vi "SSH_TUNNEL_Close.vi"(8 "error in (no error)":errorcluster, 11 "SSH_TUNNEL in":refnum<class "SSH_TUNNEL.lvclass">) -> (0 "error out":errorcluster, 3 "SSH_TUNNEL out":refnum<class "SSH_TUNNEL.lvclass">)   [LabVIEW 2018, in "SSH_TUNNEL.lvclass"]
uses:
  SSH_TUNNEL.lvclass
  SSH_TUNNEL.lvclass/SSH_TUNNEL.ctl
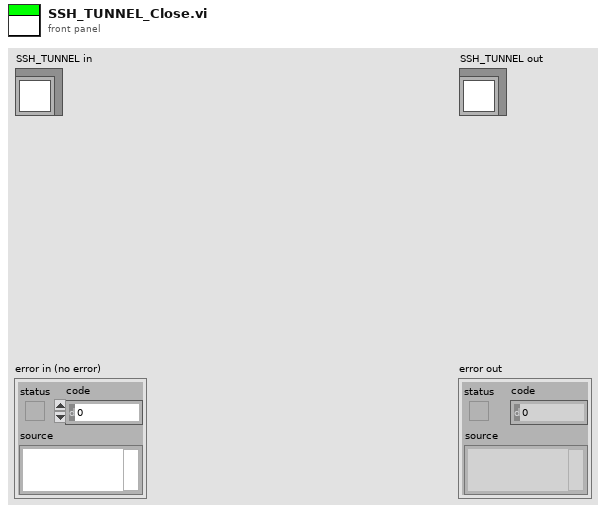
[diagram p1: front panel]
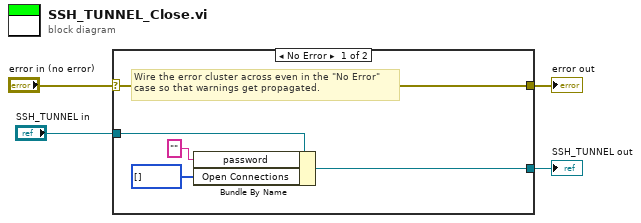
[diagram p0: block diagram]
diagram:
  n1 = case shown="No Error" "error in (no error)" {
    selector: "error in (no error)" -> [w9 w11]
    tunnel: [w9 w11] -> w3
    tunnel: [w7 w10] -> w1
    tunnel: "SSH_TUNNEL in" -> [w8 w10]
    frame No Error {
      # "Wire the error cluster across even in the \"No Error\"\ncase so that warnings get propagated."
      n2 = Bundle By Name(cluster=w8, "password"="", "Open Connections"=u16[] []) -> (w7:refnum<class "SSH_TUNNEL.lvclass">)
    }
    frame Error {
    }
  }
  "error out" <- w3
  "SSH_TUNNEL out" <- w1
